vi "Bind Text.vi"(8 "error in (no error)":errorcluster, 10 "Text":string, 11 "SQL Statement in":refnum<class "SQL Statement.lvclass">) -> (0 "error out":errorcluster, 3 "SQL Statement out":refnum<class "SQL Statement.lvclass">)   [LabVIEW 2023, in "SQLiteSupport.lvlib" / "SQL Statement.lvclass"]
doc: "Binds the next parameter as an SQLite3 TEXT datatype."
uses:
  SQL Statement.lvclass
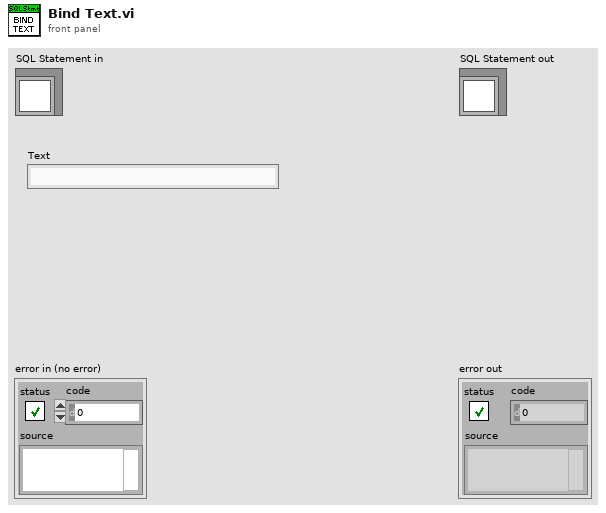
[diagram p1: front panel]
types:
  T1 = typedef "SQLiteSupport.lvlib/SQL Statement.lvclass/Text Encoding" = enum16{"System", "UTF-8", "UTF-16"}
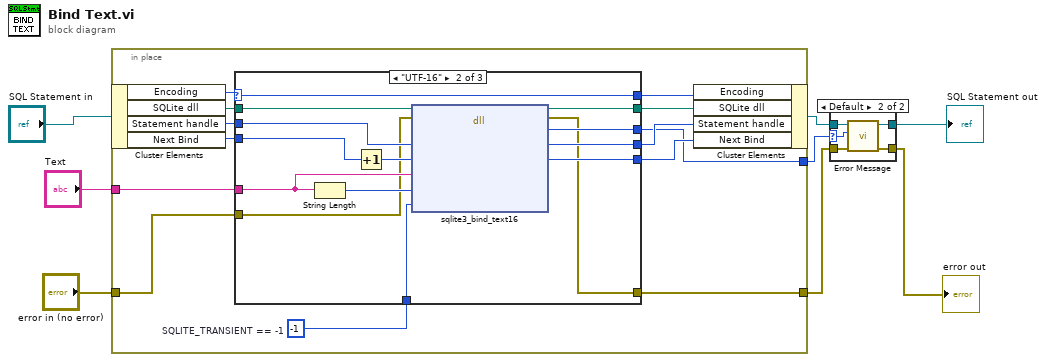
[diagram p0: block diagram]
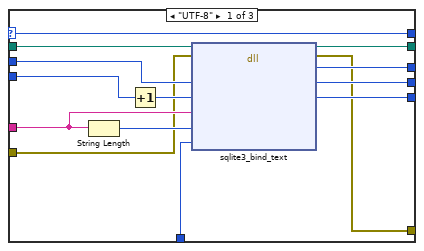
[diagram p2: hidden frame]
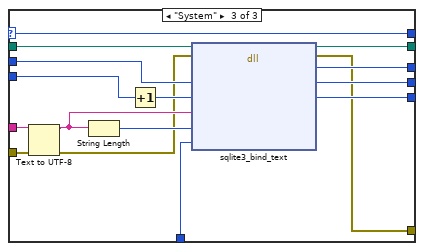
[diagram p3: hidden frame]
diagram:
  n1 = in-place {
    in-place-border: "error in (no error)" -> [w11]
    in-place-border: "Text" -> [w12]
    in-place-border: [w14] -> w2
    in-place-border: [w13] -> w1
    w21 = i64 -1  # SQLITE_TRANSIENT == -1
    n2 = in-place-cluster #1("SQL Statement in") -> ("Encoding"=w10:T1, "SQLite dll"=w20:path, "Statement handle"=w18:u64, "Next Bind"=w17:i32)
    n3 = case shown="\"UTF-16\"" w10 {
      selector: w10 -> [w22 w36 w50]
      tunnel: w21 -> [w35 w49 w65]
      tunnel: w20 -> [w33 w47 w63]
      tunnel: [w32 w46 w62] -> w19
      tunnel: w18 -> [w31 w45 w61]
      tunnel: w17 -> [w30 w44 w60]
      tunnel: [w28 w42 w58] -> w16
      tunnel: [w27 w41 w57] -> w15
      tunnel: [w26 w40 w56] -> w14
      tunnel: [w25 w39 w55] -> w13
      tunnel: w12 -> [w24 w38 w54]
      tunnel: w11 -> [w23 w37 w52]
      tunnel: [w22 w36 w50] -> w9
      frame "UTF-8" {
        n4 = String Length(string=w24) -> (length=w34:i32)
        n5 = Increment(x=w30) -> (x+1=w29:i32)
        n6 = dll-call lib="C:/LabVIEW_JDP/Support/SQLite/SQL Connection/sqlite3.dll" fn="sqlite3_bind_text"(path in=w33, error in=w23, "Statement"=w31, "Parameter"=w29, "Text"=w24, "Number of Bytes"=w34, "arg5"=w35) -> (path out=w32:path, error out=w25:errorcluster, "Result Code"=w26:i32, "Statement"=w27:u64, "Parameter"=w28:i32)  [unwired: 4 in]
      }
      frame "UTF-16" {
        n7 = String Length(string=w38) -> (length=w48:i32)
        n8 = Increment(x=w44) -> (x+1=w43:i32)
        n9 = dll-call lib="C:/LabVIEW_JDP/Support/SQLite/SQL Connection/sqlite3.dll" fn="sqlite3_bind_text16"(path in=w47, error in=w37, "Statement"=w45, "Parameter"=w43, "Text"=w38, "Number of Bytes"=w48, "arg5"=w49) -> (path out=w46:path, error out=w39:errorcluster, "Result Code"=w40:i32, "Statement"=w41:u64, "Parameter"=w42:i32)  [unwired: 4 in]
      }
      frame "System" {
        n10 = Text to UTF-8(8:w52, 11:w54) -> (0:w51:errorcluster, 3:w53:string)  [unwired: 1 in]
        n11 = String Length(string=w53) -> (length=w64:i32)
        n12 = Increment(x=w60) -> (x+1=w59:i32)
        n13 = dll-call lib="C:/LabVIEW_JDP/Support/SQLite/SQL Connection/sqlite3.dll" fn="sqlite3_bind_text"(path in=w63, error in=w51, "Statement"=w61, "Parameter"=w59, "Text"=w53, "Number of Bytes"=w64, "arg5"=w65) -> (path out=w62:path, error out=w55:errorcluster, "Result Code"=w56:i32, "Statement"=w57:u64, "Parameter"=w58:i32)  [unwired: 4 in]
      }
    }
    n14 = in-place-cluster #1("Encoding"=w9, "SQLite dll"=w19, "Statement handle"=w15, "Next Bind"=w16) -> (w3:refnum<class "SQL Statement.lvclass">)
  }
  n15 = case shown="Default" w2 {
    selector: w2 -> [_ w68]
    tunnel: w3 -> [w67 w72]
    tunnel: [w67 w71] -> w6
    tunnel: w1 -> [w66 w70]
    tunnel: [w66 w69] -> w5
    frame 0 {
      # "No Error"
    }
    frame Default {
      n16 = call "Error Message.vi"("error in (no error)"=w70, "error code"=w68, "SQL Statement In"=w72) -> ("error out"=w69:errorcluster, "SQL Statement Out"=w71:refnum<class "SQL Statement.lvclass">)  [unwired: 7 in]
    }
  }
  "error out" <- w5
  "SQL Statement out" <- w6
